vi "Send Input Data to Service VI.vi"(8 "error in (no error)":errorcluster, 10 "Data":T1, 11 "Service VI In":refnum<vi>) -> (0 "error out":errorcluster, 3 "Service VI Out":refnum<vi>)   [LabVIEW 2014]
uses:
  _typedefs/impExp_Data.ctl
  <vilib>/NI Veristand/Templates/Workspace Tool Support/Workspace Tool Message Bus.ctl
  <vilib>/NI Veristand/Templates/Workspace Tool Support/Workspace Tool Message (String).ctl
  <vilib>/NI Veristand/Templates/Workspace Tool Support/Workspace Tool Response (String).ctl
  <vilib>/NI Veristand/Templates/Workspace Tool Support/Workspace Tool Message (Byte Array).ctl
  <vilib>/NI Veristand/Templates/Workspace Tool Support/Workspace Tool Response (Byte Array).ctl
  <vilib>/NI VeriStand/Templates/Workspace Tool Support/NI VeriStand - Workspace Tool Support.lvlib
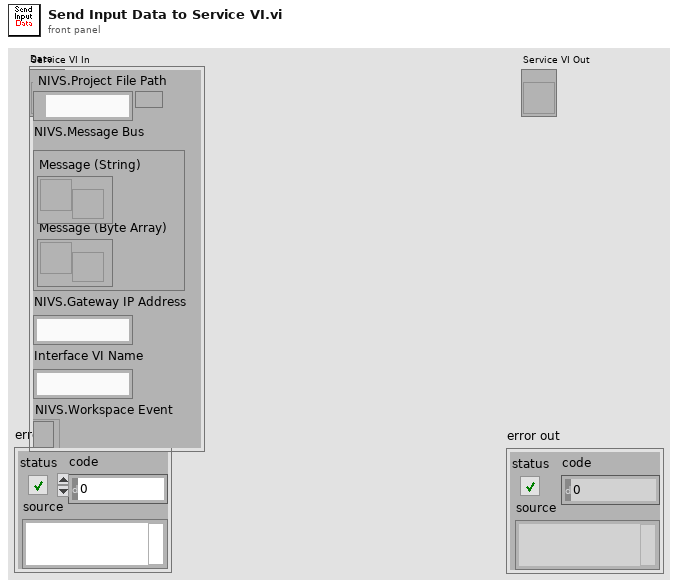
[diagram p1: front panel]
types:
  T1 = typedef "impExp_Data.ctl" = cluster{"NIVS.Project File Path":path, "NIVS.Message Bus":T2, "NIVS.Gateway IP Address":string, "Interface VI Name":string, "NIVS.Workspace Event":refnum<event-registration>}
  T2 = typedef "NI VeriStand - Workspace Tool Support.lvlib/Workspace Tool Message Bus.ctl" = cluster{"Message (String)":refnum<user-event>, "Message (Byte Array)":refnum<user-event>}
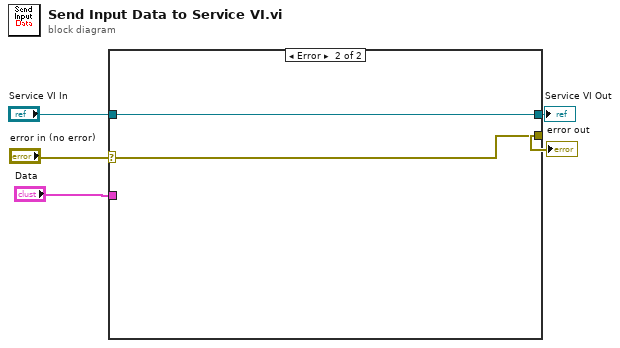
[diagram p0: block diagram]
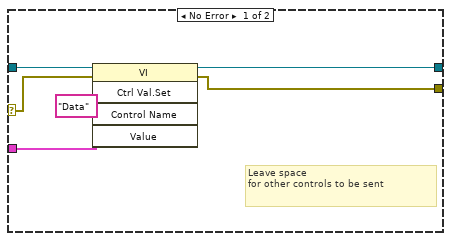
[diagram p2: hidden frame]
diagram:
  n1 = case shown="Error" "error in (no error)" {
    selector: "error in (no error)" -> [w10 w12]
    tunnel: "Service VI In" -> [w11 w13]
    tunnel: "Data" -> [w9 _]
    tunnel: [w7 w13] -> w2
    tunnel: [w6 w12] -> w1
    frame No Error {
      # "Leave space\nfor other controls to be sent"
      n2 = invoke class="VI" method="Ctrl Val.Set"(reference=w11, error in=w10, "Control Name"="Data", "Value"=w9) -> (reference out=w7:refnum<vi>, error out=w6:errorcluster)  [unwired: 1 in, 3 out]
    }
    frame Error {
    }
  }
  "Service VI Out" <- w2
  "error out" <- w1
